vi "Memory.Pointer.Error Handling.Generate Error.Offset.vi"(7 "source vi name":string, 8 "error in (no error)":errorcluster, 9 "min (0)":u64 format="%d bytes", 10 "max":u64 format="%d bytes", 11 "offset":u64 format="%d bytes") -> (0 "error out":errorcluster)   [LabVIEW 2016, in "LabVIEW Memory Manager.lvlib" / "Memory.Pointer.lvclass"]
uses:
  Memory.Pointer.lvclass
  Typedefs/Memory.Pointer.Error Codes.ctl
  RT Errors/VIs/Deterministic Errors.New Error Cluster (256B).vi
  Memory.Globals.vi
  RT Errors/Deterministic Error Builder.lvlib
  LabVIEW Memory Manager.lvlib
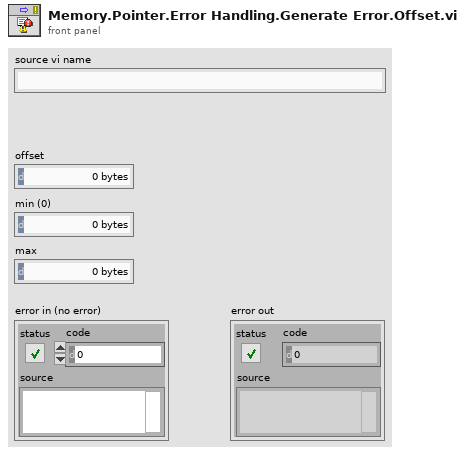
[diagram p1: front panel]
types:
  T1 = typedef "LabVIEW Memory Manager.lvlib/Memory.Pointer.lvclass/Memory.Pointer.Error Codes.ctl" = enum16{"Out of range"}
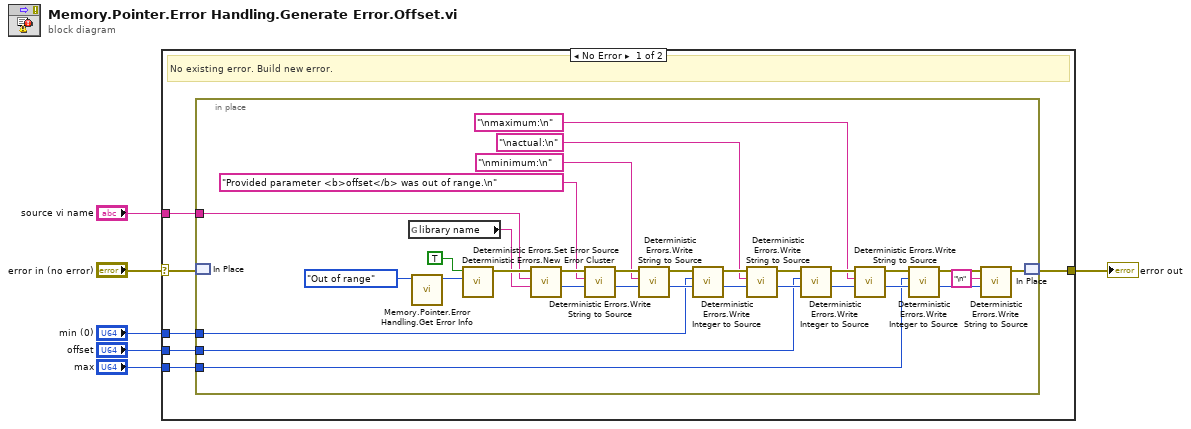
[diagram p0: block diagram]
diagram:
  n1 = case shown="No Error" "error in (no error)" {
    selector: "error in (no error)" -> [w11 w44]
    tunnel: [w12 w44] -> w1
    tunnel: "offset" -> [w9 _]
    tunnel: "min (0)" -> [w8 _]
    tunnel: "max" -> [w7 _]
    tunnel: "source vi name" -> [w10 _]
    frame No Error {
      # "No existing error. Build new error."
      n2 = in-place {
        in-place-border: w10 -> [w40]
        in-place-border: w9 -> [w28]
        in-place-border: w8 -> [w19]
        in-place-border: w7 -> [w20]
        n3 = in-place-match #1(w11) -> ()  [unwired: 1 out]
        n4 = global read "Memory.Globals.vi" "library name"() -> (w13:string)
        n5 = call "Memory.Pointer.Error Handling.Get Error Info.vi"("error"=Memory.Pointer.Error_Codes."Out of range" ("error code")) -> ("code"=w41:i32)  [unwired: 9 in, 1 out]
        n6 = call-poly "Deterministic Errors.New Error Cluster.vi"("code (0)"=w41, "status (F)"=TRUE) -> ("error out"=w43:errorcluster)  [unwired: 9 in]
        n7 = call "Deterministic Errors.Set Error Source.vi"("library name (\"\")"=w13, "vi name"=w40, "error in"=w43) -> ("new offset"=w22:i32, "error out"=w23:errorcluster)  [unwired: 7 in]
        n8 = call "Deterministic Errors.Write String to Source.vi"("offset (0)"=w22, "string"="Provided parameter <b>offset</b> was out of range.\n", "error in"=w23) -> ("new offset"=w38:i32, "error out"=w39:errorcluster)  [unwired: 7 in]
        n9 = call "Deterministic Errors.Write String to Source.vi"("offset (0)"=w38, "string"="\nminimum:\n", "error in"=w39) -> ("new offset"=w34:i32, "error out"=w37:errorcluster)  [unwired: 7 in]
        n10 = call "Deterministic Errors.Write Integer to Source.vi"("offset (0)"=w34, "value"=w19, "error in"=w37) -> ("new offset"=w35:i32, "error out"=w36:errorcluster)  [unwired: 7 in]
        n11 = call "Deterministic Errors.Write String to Source.vi"("offset (0)"=w35, "string"="\nactual:\n", "error in"=w36) -> ("new offset"=w29:i32, "error out"=w30:errorcluster)  [unwired: 7 in]
        n12 = call "Deterministic Errors.Write Integer to Source.vi"("offset (0)"=w29, "value"=w28, "error in"=w30) -> ("new offset"=w26:i32, "error out"=w27:errorcluster)  [unwired: 7 in]
        n13 = call "Deterministic Errors.Write String to Source.vi"("offset (0)"=w26, "string"="\nmaximum:\n", "error in"=w27) -> ("new offset"=w24:i32, "error out"=w25:errorcluster)  [unwired: 7 in]
        n14 = call "Deterministic Errors.Write Integer to Source.vi"("offset (0)"=w24, "value"=w20, "error in"=w25) -> ("new offset"=w14:i32, "error out"=w17:errorcluster)  [unwired: 7 in]
        n15 = call "Deterministic Errors.Write String to Source.vi"("offset (0)"=w14, "string"="\n", "error in"=w17) -> ("error out"=w16:errorcluster)  [unwired: 7 in, 1 out]
        n16 = in-place-match #1(w16) -> (w12:errorcluster)
      }
    }
    frame Error {
      # "Incoming error. Pass through."
    }
  }
  "error out" <- w1
